vi "FIFO Flush-timings.vi"() -> ()   [LabVIEW 2020]
uses:
  <vilib>/rvi/interface/nirviMethod/nirviMethod.xnode
  <vilib>/FPGAPlugInAG/Dynamic/niLvFpga_ReadFifo_Dynamic.vi
  <vilib>/rvi/errors/niLvFpgaMergeErrorWithErrorCode.vi
  RIG-SPECIFIC FILES/FPGA Refs/FPGA Ref.ctl
panel:
  in  "FPGA VI Ref":T1
  out "Data Image Time":u64[](array[numeric])
  out "Image time zero":u32
  out "Data Ref Time FIFO":u64[](array[numeric])
  out "Ref time zero":u32
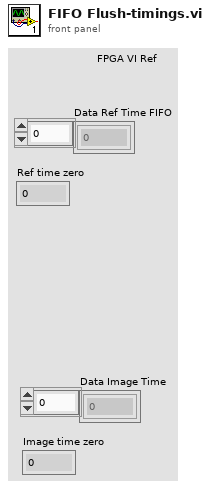
[diagram p1: front panel]
types:
  T1 = typedef "FPGA Ref.ctl" = refnum<k20>
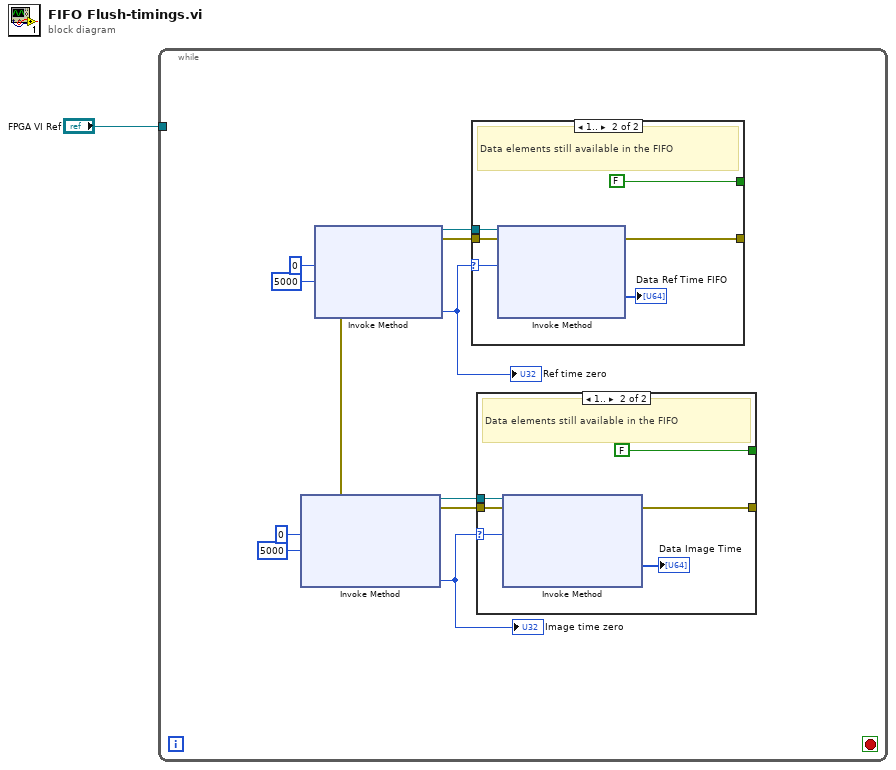
[diagram p0: block diagram]
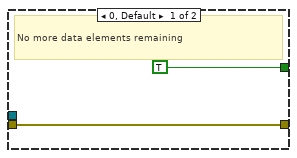
[diagram p2: hidden frame]
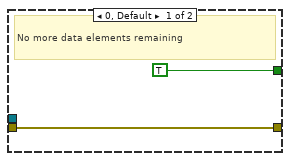
[diagram p3: hidden frame]
diagram:
  n1 = while {
    tunnel: "FPGA VI Ref" -> [_]
    stop <- _ stop-if-true
    n2 = xnode "Invoke Method"("Number of Elements"=u32 0, "Timeout (ms)"=5000) -> ("FPGA VI Reference In"=w2:refnum<k20>, "FPGA VI Reference Out"=w10:refnum<k20>, "error in"=w3:errorcluster, "error out"=w9:errorcluster, "Elements Remaining"=w13:u32)  [unwired: 1 out]
    "Ref time zero" <- w13
    n3 = xnode "Invoke Method"("FPGA VI Reference In"=w2, "error in"=w3, "Number of Elements"=u32 0, "Timeout (ms)"=5000) -> ("FPGA VI Reference Out"=w7:refnum<k20>, "error out"=w8:errorcluster, "Elements Remaining"=w4:u32)  [unwired: 1 out]
    "Image time zero" <- w4
    n4 = case shown="1.." w13 {
      selector: w13 -> [_ w26]
      tunnel: w9 -> [w22 w29]
      tunnel: w10 -> [_ w28]
      tunnel: [w22 w27] -> _
      tunnel: [TRUE FALSE] -> _
      frame 0, Default {
        # "No more data elements remaining"
      }
      frame 1.. {
        # "Data elements still available in the FIFO"
        n5 = xnode "Invoke Method"("FPGA VI Reference In"=w28, "error in"=w29, "Number of Elements"=w26) -> ("error out"=w27:errorcluster, "Data"=→"Data Ref Time FIFO":u64[])  [unwired: 1 in, 2 out]
      }
    }
    n6 = case shown="1.." w4 {
      selector: w4 -> [_ w18]
      tunnel: w8 -> [w14 w21]
      tunnel: w7 -> [_ w20]
      tunnel: [w14 w19] -> _
      tunnel: [TRUE FALSE] -> _
      frame 0, Default {
        # "No more data elements remaining"
      }
      frame 1.. {
        # "Data elements still available in the FIFO"
        n7 = xnode "Invoke Method"("FPGA VI Reference In"=w20, "error in"=w21, "Number of Elements"=w18) -> ("error out"=w19:errorcluster, "Data"=→"Data Image Time":u64[])  [unwired: 1 in, 2 out]
      }
    }
  }
